vi "Configure Marker Frequency Counter.vi"(0 "VISA resource name":refnum<visa-resource-name>, 1 "Enable Counter (T: Enable)":bool=TRUE, 2 "Enable Signal Track (T: Enable)":bool=TRUE, 5 "Active Marker (1: Marker1)":u16(ring)=1 items=["Marker1"=1, "Marker2"=2, "Marker3"=3, "Marker4"=4], 7 "Enable Auto Resolution (T: Enable)":bool=TRUE, 9 "Manual Resolution (1000 Hz)":dbl=1000.0, 11 "error in (no error)":errorcluster, 12 "Enable Auto Gate Time (T: Enable)":bool=TRUE, 13 "Manual Gate Time (100 ms)":dbl=0.1) -> (4 "VISA resource name out":refnum<visa-resource-name>, 15 "error out":errorcluster)   [LabVIEW 2014, in "Agilent ESA PSA Series.lvlib"]
doc: "Sets the marker frequency counter resolution, Gate Time and turns the marker frequency counter on/off."
uses:
  Agilent ESA PSA Series.lvlib
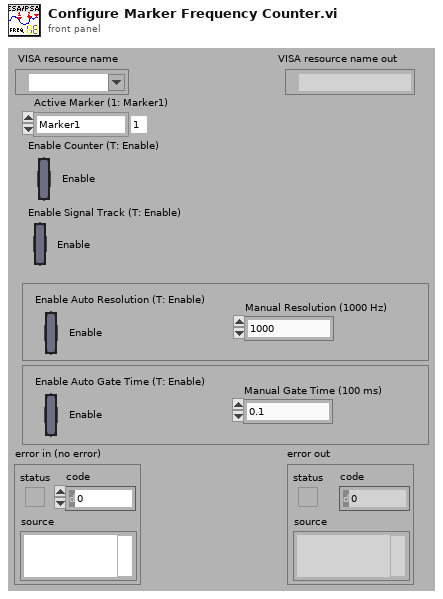
[diagram p1: front panel]
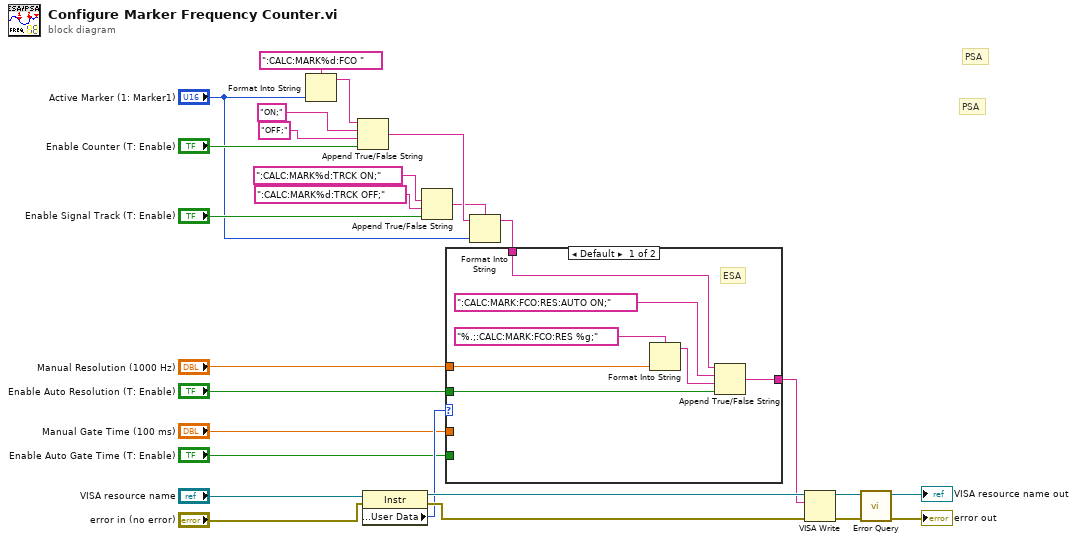
[diagram p0: block diagram]
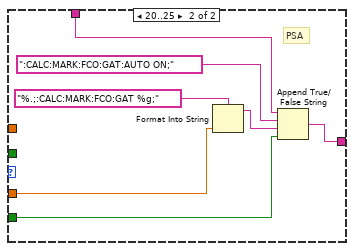
[diagram p2: hidden frame]
diagram:
  # "PSA"
  # "PSA"
  n1 = Format Into String(format string=":CALC:MARK%d:FCO ", "Active Marker (1: Marker1)") -> (resulting string=w18:string)  [unwired: 2 in, 1 out]
  n2 = Append True/False String(1:"Enable Counter (T: Enable)", 2:"OFF;" ("false string"), 3:"ON;" ("false string"), 4:w18) -> (0:w4:string)
  n3 = property on="Property Node" class="Instr"(reference="VISA resource name", error in="error in (no error)") -> (reference out=w14:refnum<visa-resource-name>, error out=w15:errorcluster, "General Settings:User Data"=w13:u32)
  n4 = Append True/False String(1:"Enable Signal Track (T: Enable)", 2:":CALC:MARK%d:TRCK OFF;" ("false string"), 3:":CALC:MARK%d:TRCK ON;" ("true string")) -> (0:w3:string)  [unwired: 1 in]
  n5 = Format Into String(format string=w3, initial string=w4, "Active Marker (1: Marker1)") -> (resulting string=w2:string)  [unwired: 1 in, 1 out]
  n6 = case shown="Default" w13 {
    tunnel: "Manual Resolution (1000 Hz)" -> [w33 _]
    tunnel: "Enable Auto Resolution (T: Enable)" -> [w29 _]
    tunnel: w2 -> [w28 w37]
    tunnel: "Manual Gate Time (100 ms)" -> [_ w36]
    tunnel: "Enable Auto Gate Time (T: Enable)" -> [_ w35]
    tunnel: [w27 w34] -> w8
    frame Default {
      # "ESA"
      n7 = Format Into String(format string="%.;:CALC:MARK:FCO:RES %g;", w33) -> (resulting string=w31:string)  [unwired: 2 in, 1 out]
      n8 = Append True/False String(1:w29, 2:w31, 3:":CALC:MARK:FCO:RES:AUTO ON;" ("initial string"), 4:w28) -> (0:w27:string)
    }
    frame 20..25 {
      # "PSA"
      n9 = Format Into String(format string="%.;:CALC:MARK:FCO:GAT %g;", w36) -> (resulting string=w39:string)  [unwired: 2 in, 1 out]
      n10 = Append True/False String(1:w35, 2:w39, 3:":CALC:MARK:FCO:GAT:AUTO ON;" ("initial string"), 4:w37) -> (0:w34:string)
    }
  }
  n11 = VISA Write(VISA resource name=w14, write buffer=w8, error in (no error)=w15) -> (VISA resource name out=w26:refnum<visa-resource-name>, error out=w24:errorcluster)  [unwired: 1 out]
  n12 = call "Error Query.vi"("error in (no error)"=w24, "VISA resource name"=w26) -> ("error out"=→"error out":errorcluster, "VISA resource name out"=→"VISA resource name out":refnum<visa-resource-name>)  [unwired: 6 in, 2 out]
